vi "Measure.vi"(8 "error in":errorcluster, 11 "Instruments in":refnum<class "Instruments.lvclass">) -> (0 "error out":errorcluster, 3 "Instruments out":refnum<class "Instruments.lvclass">)   [LabVIEW 2023, in "Instruments.lvlib" / "Instruments.lvclass"]
uses:
  Library/Instruments.lvclass
  C:/Users/Public/Documents/Development/builds/Engine/Engine.lvlibp/Project/Engine.lvclass
  C:/Users/Public/Documents/Development/builds/Engine/Actor Framework.lvlibp/1abvi3w/vi.lib/ActorFramework/Actor/Actor.lvclass
  Library/Instruments.lvclass/Instruments.ctl
  builds/Engine/Engine.lvlibp/Accessors/Read Report Queue.vi
  builds/Engine/Actor Framework.lvlibp/1abvi3w/vi.lib/ActorFramework/Actor/Read Actor Label.vi
  builds/Tools/QDMH.lvlibp/Private/Enqueue Bundled Element.vi
  builds/Tools/QDMH.lvlibp/QDMH.lvclass
  builds/Engine/Engine.lvlibp/Project/Engine.lvclass
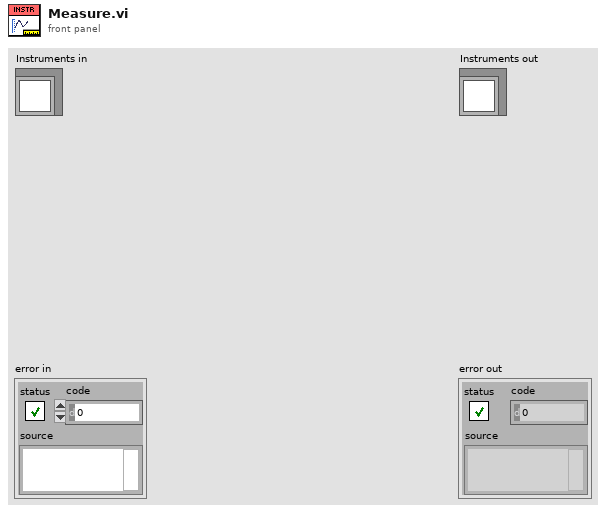
[diagram p1: front panel]
types:
  T1 = cluster{"Accessors:Actor Label":string, "Measured":waveform(dbl)[]}
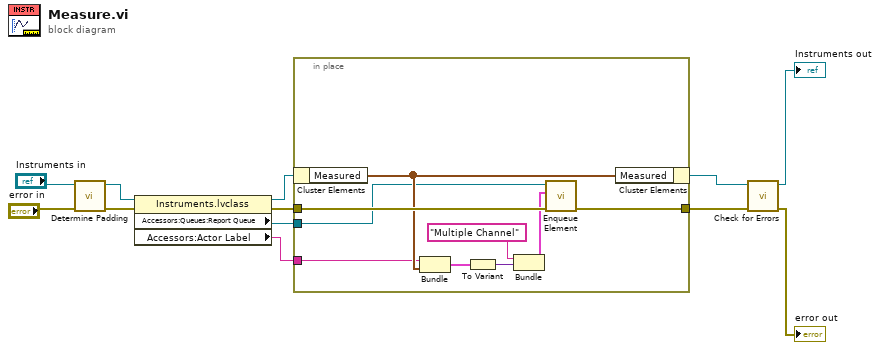
[diagram p0: block diagram]
diagram:
  n1 = call "Determine Padding.vi"("error in"="error in", "Instruments in"="Instruments in") -> ("error out"=w8:errorcluster, "Instruments out"=w7:refnum<class "Instruments.lvclass">)  [unwired: 8 in]
  n2 = property class="Instruments.lvclass"(reference=w7, error in=w8) -> (reference out=w10:refnum<class "Instruments.lvclass">, error out=w9:errorcluster, "Accessors:Queues:Report Queue"=w11:refnum<class "QDMH.lvclass">, "Accessors:Actor Label"=w12:string)
  n3 = in-place {
    in-place-border: w9 -> [w21]
    in-place-border: [w20] -> w6
    in-place-border: w11 -> [w14]
    in-place-border: w12 -> [w13]
    n4 = in-place-cluster #1(w10) -> ("Measured"=w15:waveform(dbl)[])
    n5 = Bundle("Accessors:Actor Label"=w13, "Measured"=w15) -> (w16:T1)  [unwired: 1 in]
    n6 = To Variant(anything=w16) -> (Variant=w19:variant)
    n7 = Bundle("Multiple Channel", "Variant"=w19) -> (w18:cluster{string, "Variant":variant})  [unwired: 1 in]
    n8 = call-poly "Enqueue Element.vi"("error in"=w21, "element"=w18, "QDMH in"=w14) -> ("error out"=w20:errorcluster)  [unwired: 7 in, 1 out]
    n9 = in-place-cluster #1("Measured"=w15) -> (w5:refnum<class "Instruments.lvclass">)
  }
  n10 = call "Check for Errors.vi"("error in"=w6, "Engine in"=w5) -> ("error out"=→"error out":errorcluster, "Engine out"=→"Instruments out":refnum<class "Instruments.lvclass">)  [unwired: 8 in]
